vi "probe_pol.vi"() -> ()   [LabVIEW 2011]
uses:
  <vilib>/express/express shared/transition.llb/Dynamic To Waveform Array.vi
  <vilib>/express/express shared/transition.llb/Waveform Array To Dynamic.vi
  <vilib>/express/express arith-compare/Formula/Block/exnFormulaBlock how many pts in the wave.vi
  <vilib>/express/express shared/ex_Modify Signal Name.vi
  <vilib>/express/express arith-compare/Formula/XNode/ExpressFormulaBlockNode.xnode
panel:
  out "M_ratio":dbl
  out "Right Peak to Peak":dbl
  out "Right DC":dbl
  out "Left Peak to Peak":dbl
  out "Left DC":dbl
  out "Right Ratio":dbl
  out "Left Ratio":dbl
  in  "Shutter":bool
  out "r at zero pol":dbl
  out "r":dbl
  in  "Number Right Samples":i32=1100
  in  "Set Magnet Off Levels":bool
  out "Right Discharge On, Magnet Off":dbl
  out "Left Discharge On, Magnet Off":dbl
  out "Waveform Chart":dynamicdata(graph)
  out "Polarization":dbl
  in  "Set Discharge Off Levels":bool
  out "Right Discharge Off":dbl
  out "Left Discharge Off":dbl
  in  "Number Left Samples":i32=2000
  out "Right Mean":dbl
  out "Left Mean":dbl
  out "Signals":dynamicdata(graph) caption="Section"
  in  "High Signal Start":i32=100 caption="Begin Sample"
  in  "Low Signal Start":i32=1000 caption="Begin Sample"
  in  "stop":bool
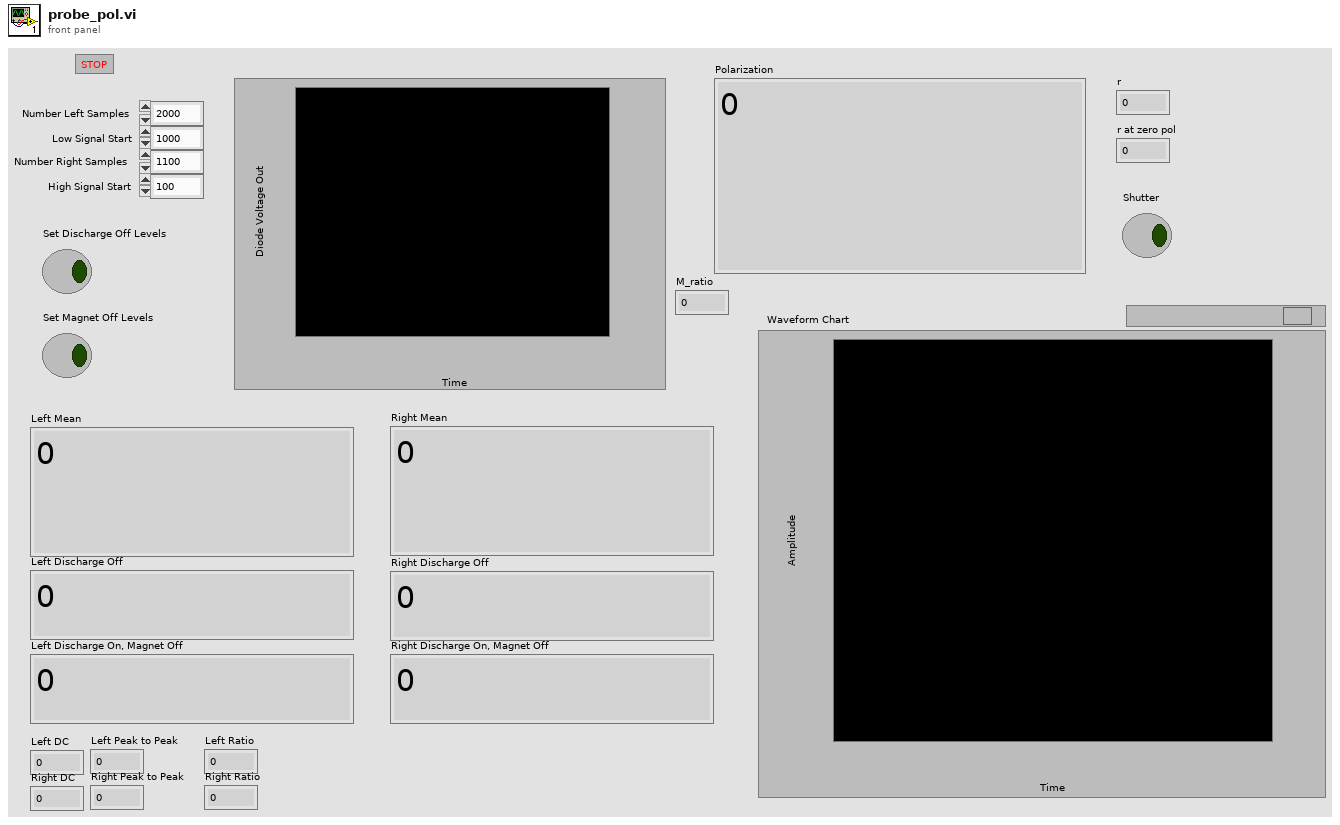
[diagram p1: front panel]
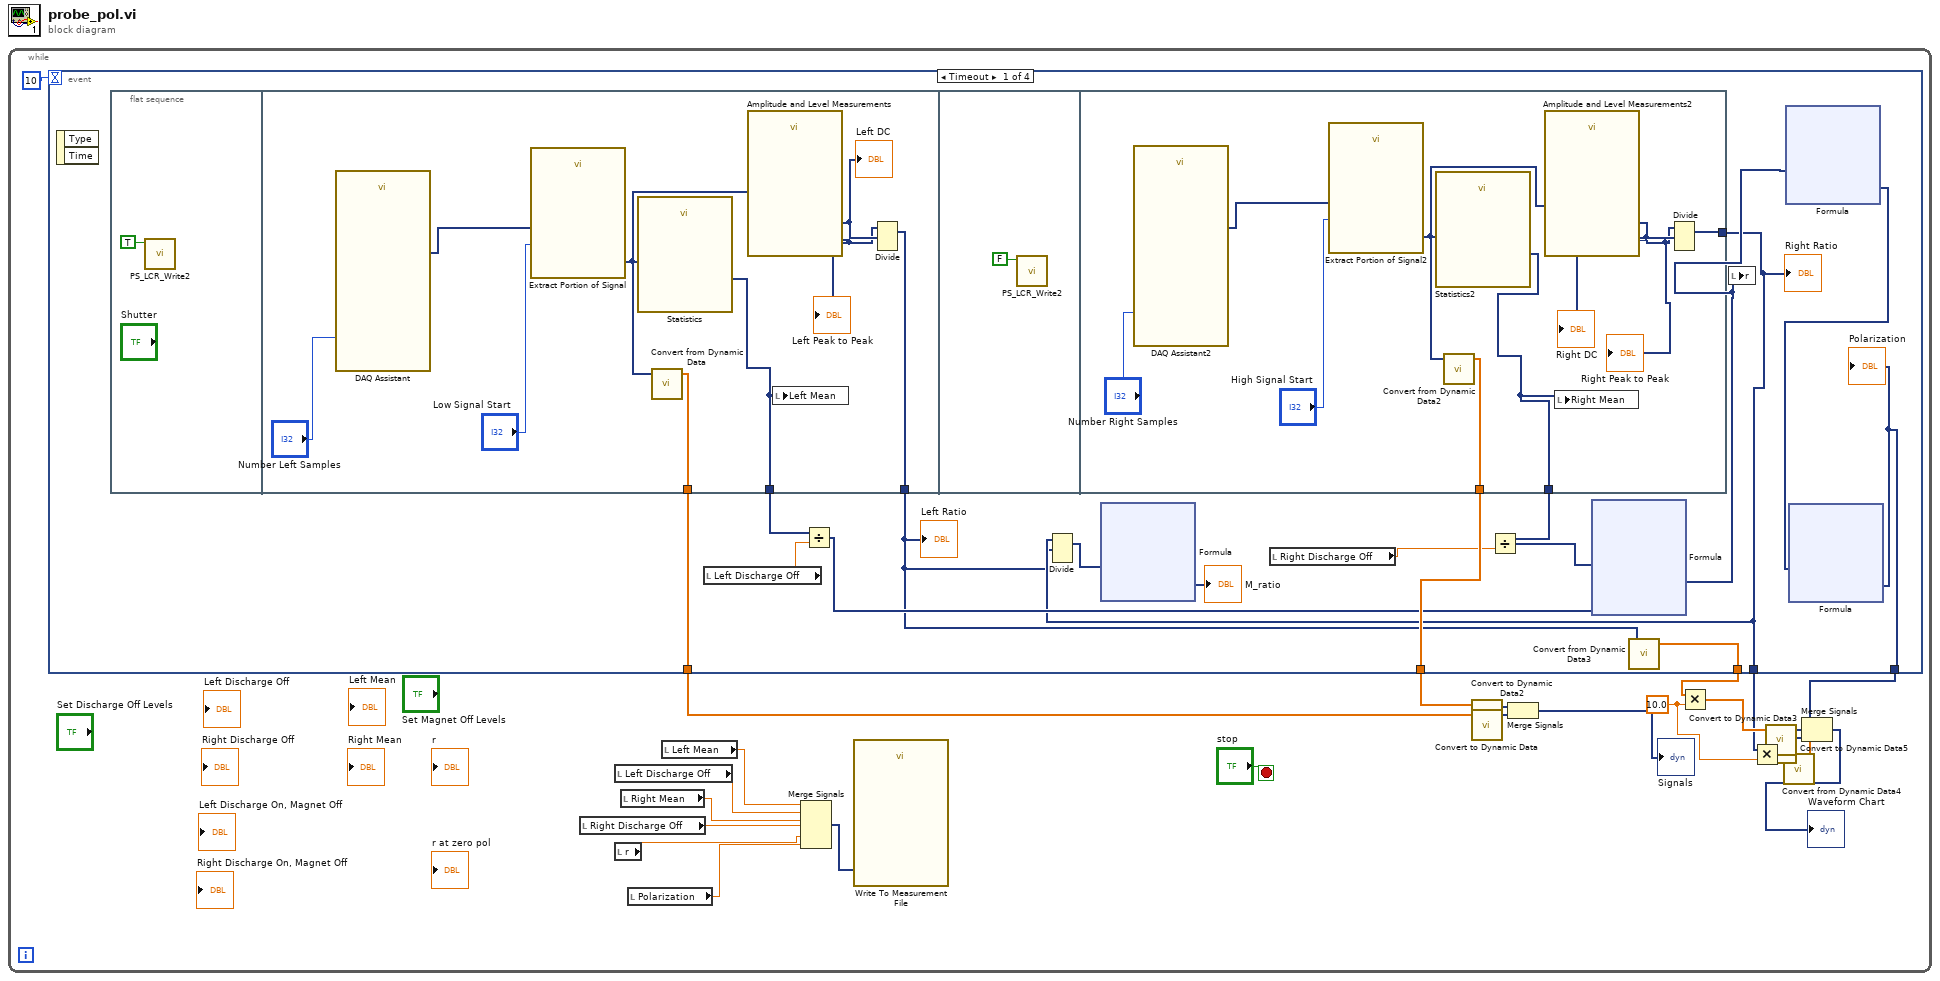
[diagram p0: block diagram]
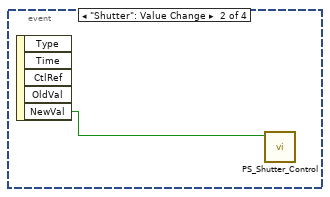
[diagram p2: hidden frame]
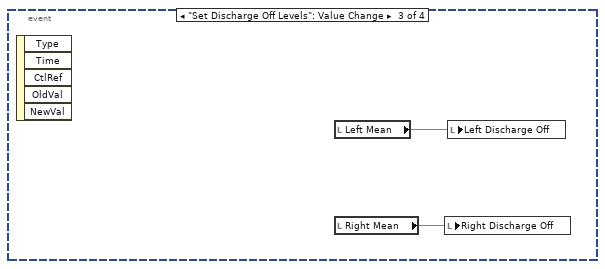
[diagram p3: hidden frame]
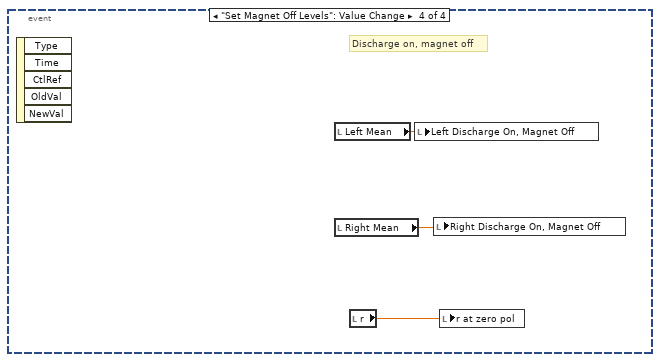
[diagram p4: hidden frame]
diagram:
  n1 = while {
    stop <- "stop" stop-if-true
    w6 = 10.0 ("y")
    n2 = event shown="[0] Timeout" {
      selector: _ -> [_ _ _ _]
      dyn-events: _ -> [_ _ _ _]
      timeout: 10 -> [_ _ _ _]
      tunnel: [w40 _ _ _] -> w22
      tunnel: [w39 _ _ _] -> w20
      tunnel: [w32 _ _ _] -> w17
      tunnel: [w29 _ _ _] -> w8
      tunnel: [w28 _ _ _] -> w3
      event Timeout {
        n3 = event-data() -> ()  [unwired: 1 in, 2 out]
        n4 = flat-sequence {
          tunnel: [w603] -> w40
          tunnel: [w602] -> w38
          tunnel: [w598] -> w27
          tunnel: [w614] -> w39
          tunnel: [w613] -> w37
          tunnel: [w610] -> w28
          frame #0 {
            n5 = call "PS_LCR_Write2.vi"("On/Off"=TRUE) -> ()  [unwired: 10 in, 1 out]
          }
          frame #1 {
            n6 = call "DAQ Assistant"("number of samples"="Number Left Samples") -> ("data"=w605:dynamicdata)  [unwired: 16 in, 2 out]
            n7 = call "Extract Portion of Signal"("Begin Sample"="Low Signal Start", "Signals"=w605) -> ("Section"=w601:dynamicdata)  [unwired: 8 in, 1 out]
            n8 = call "Statistics"("Signals"=w601) -> ("Arithmetic Mean"=w602:dynamicdata)  [unwired: 24 in, 2 out]
            n9 = call "Convert from Dynamic Data"("Dynamic Data Type"=w601) -> ("Array"=w603:dbl[])  [unwired: 3 in]
            n10 = call "Amplitude and Level Measurements"("Signals"=w601) -> ("Mean (DC)"=w600:dynamicdata, "Peak to Peak"=w599:dynamicdata)  [unwired: 12 in, 1 out]
            "Left DC" <- w600
            "Left Peak to Peak" <- w599
            n11 = local write "Left Mean"(w602) -> ()
            n12 = Divide(1:w600, 2:w599) -> (0:w598:dynamicdata)  [unwired: 1 in, 1 out]
          }
          frame #2 {
            n13 = call "PS_LCR_Write2.vi"("On/Off"=FALSE) -> ()  [unwired: 10 in, 1 out]
          }
          frame #3 {
            n14 = call "DAQ Assistant2"("number of samples"="Number Right Samples") -> ("data"=w615:dynamicdata)  [unwired: 16 in, 2 out]
            n15 = call "Extract Portion of Signal2"("Begin Sample"="High Signal Start", "Signals"=w615) -> ("Section"=w611:dynamicdata)  [unwired: 8 in, 1 out]
            n16 = call "Statistics2"("Signals"=w611) -> ("Arithmetic Mean"=w613:dynamicdata)  [unwired: 24 in, 2 out]
            n17 = call "Convert from Dynamic Data2"("Dynamic Data Type"=w611) -> ("Array"=w614:dbl[])  [unwired: 3 in]
            n18 = call "Amplitude and Level Measurements2"("Signals"=w611) -> ("Mean (DC)"=w609:dynamicdata, "Peak to Peak"=w608:dynamicdata)  [unwired: 12 in, 1 out]
            "Right DC" <- w609
            "Right Peak to Peak" <- w608
            n19 = local write "Right Mean"(w613) -> ()
            n20 = Divide(1:w609, 2:w608) -> (0:w610:dynamicdata)  [unwired: 1 in, 1 out]
          }
        }
        n21 = local read "Left Discharge Off"() -> (w36:dbl)
        n22 = Divide(x=w38, y=w36) -> (x/y=w33:dynamicdata)
        n23 = Divide(1:w27, 2:w28) -> (0:w26:dynamicdata)  [unwired: 1 in, 1 out]
        n24 = xnode "Formula"("r"=w26) -> ("Result"=→"M_ratio":dynamicdata)  [unwired: 1 in, 1 out]
        n25 = local read "Right Discharge Off"() -> (w35:dbl)
        n26 = Divide(x=w37, y=w35) -> (x/y=w34:dynamicdata)
        n27 = xnode "Formula"("Ar"=w34, "Al"=w33) -> ("Result"=w31:dynamicdata)  [unwired: 1 in, 1 out]
        n28 = call "Convert from Dynamic Data3"("Dynamic Data Type"=w27) -> ("Array"=w29:dbl[])  [unwired: 3 in]
        n29 = local write "r"(w31) -> ()
        n30 = xnode "Formula"("X1"=w31) -> ("Result"=w30:dynamicdata)  [unwired: 1 in, 1 out]
        n31 = xnode "Formula"("r"=w30) -> ("Result"=w32:dynamicdata)  [unwired: 1 in, 1 out]
        "Polarization" <- w32
        "Left Ratio" <- w27
        "Right Ratio" <- w28
      }
      event "Shutter": Value Change {
        n32 = event-data() -> ("NewVal"=w617:bool)  [unwired: 1 in, 4 out]
        n33 = call "PS_Shutter_Control.vi"("On/Off"=w617) -> ()  [unwired: 10 in, 1 out]
      }
      event "Set Discharge Off Levels": Value Change {
        n34 = event-data() -> ()  [unwired: 1 in, 5 out]
        n35 = local read "Left Mean"() -> (w619:dbl)
        n36 = local read "Right Mean"() -> (w618:dbl)
        n37 = local write "Right Discharge Off"(w618) -> ()
        n38 = local write "Left Discharge Off"(w619) -> ()
      }
      event "Set Magnet Off Levels": Value Change {
        # "Discharge on, magnet off"
        n39 = event-data() -> ()  [unwired: 1 in, 5 out]
        n40 = local read "Left Mean"() -> (w622:dbl)
        n41 = local read "Right Mean"() -> (w621:dbl)
        n42 = local read "r"() -> (w620:dbl)
        n43 = local write "Left Discharge On, Magnet Off"(w622) -> ()
        n44 = local write "Right Discharge On, Magnet Off"(w621) -> ()
        n45 = local write "r at zero pol"(w620) -> ()
      }
    }
    n46 = local read "Right Discharge Off"() -> (w12:dbl)
    n47 = local read "Left Discharge Off"() -> (w14:dbl)
    n48 = local read "r"() -> (w11:dbl)
    n49 = local read "Right Mean"() -> (w13:dbl)
    n50 = local read "Polarization"() -> (w10:dbl)
    n51 = local read "Left Mean"() -> (w15:dbl)
    n52 = Merge Signals(w15, w14, w13, w12, w11, w10) -> (w16:dynamicdata)
    n53 = call "Write To Measurement File"("Signals"=w16) -> ()  [unwired: 16 in, 3 out]
    n54 = call "Convert to Dynamic Data2"("Array"=w20) -> ("Dynamic Data Type"=w19:dynamicdata)  [unwired: 3 in]
    n55 = call "Convert to Dynamic Data"("Array"=w22) -> ("Dynamic Data Type"=w21:dynamicdata)  [unwired: 3 in]
    n56 = Merge Signals(w19, w21) -> (→"Signals":dynamicdata)
    n57 = Multiply(x=w8, y=w6) -> (x*y=w7:dbl[])
    n58 = Multiply(x=w3, y=w6) -> (x*y=w2:dynamicdata)
    n59 = call "Convert to Dynamic Data3"("Array"=w7) -> ("Dynamic Data Type"=w5:dynamicdata)  [unwired: 3 in]
    n60 = call "Convert from Dynamic Data4"("Dynamic Data Type"=w2) -> ("Array"=w1:dbl[])  [unwired: 3 in]
    n61 = call "Convert to Dynamic Data5"("Array"=w1) -> ("Dynamic Data Type"=w4:dynamicdata)  [unwired: 3 in]
    n62 = Merge Signals(w17, w5, w4) -> (→"Waveform Chart":dynamicdata)
  }
